vi "Edit Current source.vi"(8 "error in (no error)":errorcluster, 11 "Instrument parameters in":T4) -> (0 "error out":errorcluster, 3 "Instrument parameters out":T4)   [LabVIEW 2025, in "My Current Source.lvlib"]
uses:
  My Current Source.lvlib
  KE622x -- Current Range.ctl
  KE622x -- Current Ranges.ctl
  KE622x -- Output Low Connection.ctl
  KE622x -- Instrument Type.ctl
  KE622x -- On Off Control.ctl
panel:
  in  "Update?":bool
  in  "Voltage limit (V)":dbl format="%#_13g"
  in  "Output Low Connection":T1
  in  "Current Range In":T2={"Auto Range?"=TRUE, "Man / Selected\nRange"=enum."2nA"}
  # "Current source: Settings"
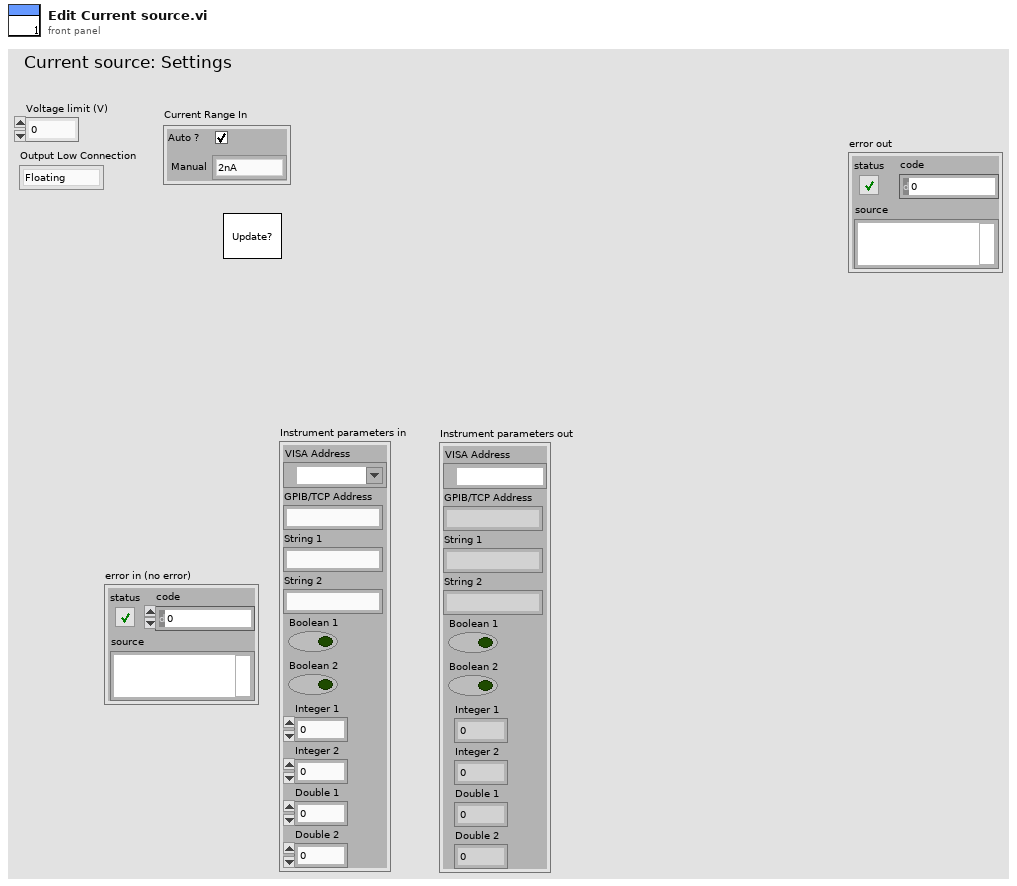
[diagram p1: front panel]
types:
  T1 = typedef "My Current Source.lvlib/KE622x -- Output Low Connection.ctl" = enum16{"Floating", "Earth Ground"}
  T2 = typedef "My Current Source.lvlib/KE622x -- Current Range.ctl" = cluster{"Auto Range?":bool, "Man / Selected\nRange":T3}
  T3 = typedef "My Current Source.lvlib/KE622x -- Current Ranges.ctl" = enum16{"2nA", "20nA", "200nA", "2uA", "20uA", "200uA", "2mA", "20mA", "100mA"}
  T4 = cluster{"VISA Address":refnum<visa-resource-name>, "GPIB/TCP Address":string, "String 1":string, "String 2":string, "Boolean 1":bool, "Boolean 2":bool, "Integer 1":i32, "Integer 2":i32, "Double 1":dbl, "Double 2":dbl}
  T5 = typedef "My Current Source.lvlib/KE622x -- On Off Control.ctl" = enum16{"Off", "On"}
  T6 = typedef "My Current Source.lvlib/KE622x -- Instrument Type.ctl" = enum16{"KE6220", "KE6221"}
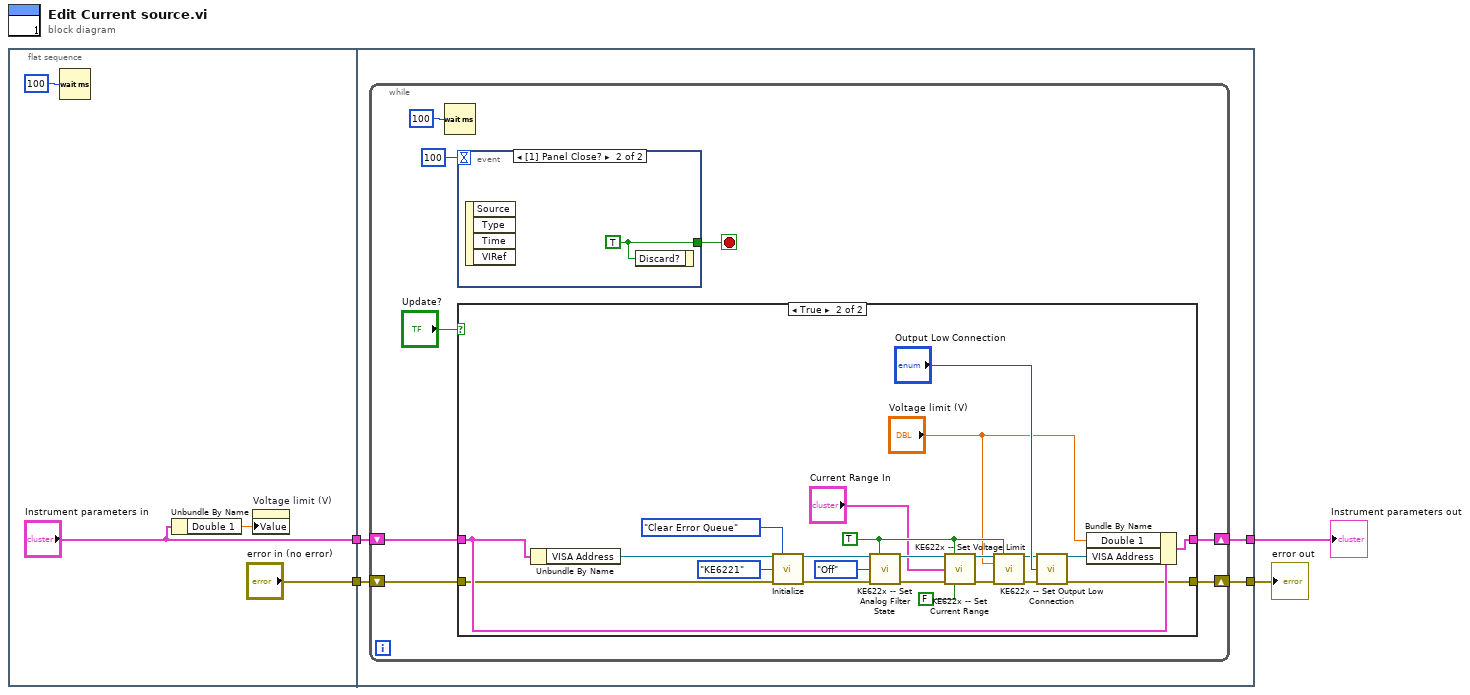
[diagram p0: block diagram]
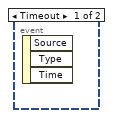
[diagram p3: hidden frame]
diagram:
  n1 = flat-sequence {
    tunnel: ["Instrument parameters in"] -> w4
    tunnel: ["error in (no error)"] -> w2
    tunnel: w4 -> [w12]
    tunnel: [w11] -> w3
    tunnel: w2 -> [w10]
    tunnel: [w9] -> w1
    frame #0 {
      n2 = Wait (ms)(milliseconds to wait=u32 100) -> ()  [unwired: 1 out]
      n3 = Unbundle By Name("Instrument parameters in") -> ("Double 1"=w6:dbl)
      n4 = property on="Voltage limit (V)" class="DigNum (strict)"("Value"=w6) -> ()  [unwired: 2 in, 2 out]
    }
    frame #1 {
      n5 = while {
        shift-right: [w18] -> w11
        shift-left: w12 -> [w19]
        shift-right: [w14] -> w9
        shift-left: w10 -> [w17]
        stop <- w16 stop-if-true
        n6 = Wait (ms)(milliseconds to wait=u32 100) -> ()  [unwired: 1 out]
        n7 = event shown="[1] Panel Close?" {
          selector: _ -> [_ _]
          dyn-events: _ -> [_ _]
          timeout: 100 -> [_ _]
          tunnel: [_ w45] -> w16
          event Timeout {
            n8 = event-data() -> ()  [unwired: 1 in, 3 out]
          }
          event Panel Close? {
            w45 = TRUE ("Discard?")
            n9 = event-data() -> ()  [unwired: 1 in, 4 out]
            n10 = event-data("Discard?"=w45) -> ()  [unwired: 1 in, 1 out]
          }
        }
        n11 = case shown="True" "Update?" {
          tunnel: w19 -> [w22 w33]
          tunnel: [w22 w32] -> w18
          tunnel: w17 -> [w21 w31]
          tunnel: [w21 w25] -> w14
          frame False {
          }
          frame True {
            w41 = TRUE ("Check For SCPI Errors? (T)")
            n12 = Unbundle By Name(w33) -> ("VISA Address"=w34:refnum<visa-resource-name>)
            n13 = call "Initialize.vi"("VISA resource name"=w34, "Error Queue Option"=enum16{"Clear Error Queue", "Error Query"}."Clear Error Queue", "Instrument Type"=KE622x_--_Instrument_Type."KE6221", "error in (no error)"=w31) -> ("VISA resource name out"=w37:refnum<visa-resource-name>, "error out"=w38:errorcluster)  [unwired: 10 in]
            n14 = call "KE622x -- Set Analog Filter State.vi"("Resource In"=w37, "Check For SCPI Errors? (T)"=w41, "Analog Filter State"=KE622x_--_On_Off_Control."Off", "error in (no error)"=w38) -> ("Resource Out (dupl)"=w30:refnum<visa-resource-name>, "error out"=w29:errorcluster)  [unwired: 10 in]
            n15 = call "KE622x -- Set Current Range.vi"("Resource In"=w30, "Check For SCPI Errors? (T)"=w41, "Current Range In"="Current Range In", "error in (no error)"=w29, "Read Back Set Values? (T)"=FALSE) -> ("Resource Out (dupl)"=w28:refnum<visa-resource-name>, "error out"=w27:errorcluster)  [unwired: 8 in, 1 out]
            n16 = call "KE622x -- Set Voltage Limit.vi"("Resource In"=w28, "Check For SCPI Errors? (T)"=w41, "Voltage limit (V)"="Voltage limit (V)", "error in (no error)"=w27) -> ("Resource Out (dupl)"=w42:refnum<visa-resource-name>, "error out"=w43:errorcluster)  [unwired: 10 in]
            n17 = call "KE622x -- Set Output Low Connection.vi"("Resource In"=w42, "Output Low Connection"="Output Low Connection", "error in (no error)"=w43) -> ("Resource Out (dupl)"=w26:refnum<visa-resource-name>, "error out"=w25:errorcluster)  [unwired: 11 in]
            n18 = Bundle By Name(cluster=w33, "Double 1"="Voltage limit (V)", "VISA Address"=w26) -> (w32:T4)
          }
        }
      }
    }
  }
  "Instrument parameters out" <- w3
  "error out" <- w1
